vi "HandleObservationSync.vi"(8 "error in (no error)":errorcluster, 11 "S4GUI in":refnum<class "S4GUI.lvclass">) -> (0 "error out":errorcluster, 3 "S4GUI out":refnum<class "S4GUI.lvclass">)   [LabVIEW 2018, in "S4GUI.lvclass"] (continued)
          n221 = call "Read Instrument.lvclass.vi"("error in (no error)"=w570, "S4ACS_GUI in"=w571) -> ("error out"=w541:errorcluster, "Instrument.lvclass"=w542:refnum<class "Instrument.lvclass">, "S4ACS_GUI out"=w572:refnum<class "S4GUI.lvclass">)  [unwired: 7 in]
          n222 = disable-structure shown="Enabled" {
            disable-tunnel: w542 -> [w576 w589]
            disable-tunnel: w541 -> [w575 w588]
            disable-tunnel: [w574 w589] -> w540
            disable-tunnel: [w573 w588] -> w539
            frame Disabled {
              n223 = call "Read WPROT.vi"("error in (no error)"=w575, "Instrument in"=w576) -> ("error out"=w579:errorcluster, "Opt_Selector.lvclass"=w580:refnum<class "Opt_Selector.lvclass">, "Instrument out"=w586:refnum<class "Instrument.lvclass">)  [unwired: 7 in]
              n224 = call-dynamic "Read State Machine.vi"("error in (no error)"=w579, "Device in"=w580) -> ("error out"=w582:errorcluster, "State Machine.lvclass"=w584:refnum<class "State Machine.lvclass">, "Device out"=w581:refnum<class "Opt_Selector.lvclass">)  [unwired: 7 in]
              n225 = call "Next State.vi"("error in (no error)"=w582, "New_State"=30, "State Machine in"=w584) -> ("error out"=w578:errorcluster, "State Machine out"=w577:refnum<class "State Machine.lvclass">)  [unwired: 7 in]
              n226 = call-dynamic "Write State Machine.vi"("error in (no error)"=w578, "State Machine.lvclass"=w577, "Device in"=w581) -> ("error out"=w585:errorcluster, "Device out"=w587:refnum<class "Opt_Selector.lvclass">)  [unwired: 7 in]
              n227 = call "Write WPROT.vi"("error in (no error)"=w585, "Opt_Selector.lvclass"=w587, "Instrument in"=w586) -> ("error out"=w573:errorcluster, "Instrument out"=w574:refnum<class "Instrument.lvclass">)  [unwired: 7 in]
            }
            frame Enabled {
              # "depois do homing no WPSEL, o homing do WPROT é feito automaticamente pelo ICS"
            }
          }
          n228 = call "Read ASEL.vi"("error in (no error)"=w539, "Instrument in"=w540) -> ("error out"=w556:errorcluster, "Opt_Selector.lvclass"=w557:refnum<class "Opt_Selector.lvclass">, "Instrument out"=w563:refnum<class "Instrument.lvclass">)  [unwired: 7 in]
          n229 = call-dynamic "Read State Machine.vi"("error in (no error)"=w556, "Device in"=w557) -> ("error out"=w559:errorcluster, "State Machine.lvclass"=w561:refnum<class "State Machine.lvclass">, "Device out"=w558:refnum<class "Opt_Selector.lvclass">)  [unwired: 7 in]
          n230 = call "Next State.vi"("error in (no error)"=w559, "New_State"=30, "State Machine in"=w561) -> ("error out"=w555:errorcluster, "State Machine out"=w554:refnum<class "State Machine.lvclass">)  [unwired: 7 in]
          n231 = call-dynamic "Write State Machine.vi"("error in (no error)"=w555, "State Machine.lvclass"=w554, "Device in"=w558) -> ("error out"=w562:errorcluster, "Device out"=w564:refnum<class "Opt_Selector.lvclass">)  [unwired: 7 in]
          n232 = Increment(x=w565) -> (x+1=w567:u32)
          n233 = call "Write ASEL.vi"("error in (no error)"=w562, "Opt_Selector.lvclass"=w564, "Instrument in"=w563) -> ("error out"=w537:errorcluster, "Instrument out"=w538:refnum<class "Instrument.lvclass">)  [unwired: 7 in]
          n234 = call "Read GMIR.vi"("error in (no error)"=w537, "Instrument in"=w538) -> ("error out"=w545:errorcluster, "Opt_Continuous.lvclass"=w546:refnum<class "Opt_Continuous.lvclass">, "Instrument out"=w552:refnum<class "Instrument.lvclass">)  [unwired: 7 in]
          n235 = call-dynamic "Read State Machine.vi"("error in (no error)"=w545, "Device in"=w546) -> ("error out"=w548:errorcluster, "State Machine.lvclass"=w550:refnum<class "State Machine.lvclass">, "Device out"=w547:refnum<class "Opt_Continuous.lvclass">)  [unwired: 7 in]
          n236 = call "Next State.vi"("error in (no error)"=w548, "New_State"=30, "State Machine in"=w550) -> ("error out"=w544:errorcluster, "State Machine out"=w543:refnum<class "State Machine.lvclass">)  [unwired: 7 in]
          n237 = call-dynamic "Write State Machine.vi"("error in (no error)"=w544, "State Machine.lvclass"=w543, "Device in"=w547) -> ("error out"=w551:errorcluster, "Device out"=w553:refnum<class "Opt_Continuous.lvclass">)  [unwired: 7 in]
          n238 = call "Write GMIR.vi"("error in (no error)"=w551, "Opt_Continuous.lvclass"=w553, "Instrument in"=w552) -> ("error out"=w536:errorcluster, "Instrument out"=w535:refnum<class "Instrument.lvclass">)  [unwired: 7 in]
          n239 = call "Write Instrument.lvclass.vi"("error in (no error)"=w536, "Instrument.lvclass"=w535, "S4ACS_GUI in"=w572) -> ("error out"=w569:errorcluster, "S4ACS_GUI out"=w568:refnum<class "S4GUI.lvclass">)  [unwired: 7 in]
          n240 = Bundle By Name(cluster=w568, "Obs_state"=w567) -> (w566:refnum<class "S4GUI.lvclass">)
        }
        frame 223 {
          # "Espera terminar o homing de WPROT,ASEL e GFOC\nantes de seguir para o próximo estado."
          n241 = call "Read Instrument.lvclass.vi"("error in (no error)"=w614, "S4ACS_GUI in"=w615) -> ("error out"=w600:errorcluster, "Instrument.lvclass"=w601:refnum<class "Instrument.lvclass">, "S4ACS_GUI out"=w609:refnum<class "S4GUI.lvclass">)  [unwired: 7 in]
          n242 = call "Read ASEL.vi"("error in (no error)"=w600, "Instrument in"=w601) -> ("error out"=w605:errorcluster, "Opt_Selector.lvclass"=w591:refnum<class "Opt_Selector.lvclass">)  [unwired: 7 in, 1 out]
          n243 = call "Read GMIR.vi"("error in (no error)"=w600, "Instrument in"=w601) -> ("error out"=w602:errorcluster, "Opt_Continuous.lvclass"=w590:refnum<class "Opt_Continuous.lvclass">)  [unwired: 7 in, 1 out]
          n244 = disable-structure shown="Enabled" {
            disable-tunnel: [w619 w625] -> w608
            disable-tunnel: w601 -> [w618 _]
            disable-tunnel: w600 -> [w617 w625]
            disable-tunnel: [w616 0 ("State")] -> w599
            frame Disabled {
              n245 = call "Read WPROT.vi"("error in (no error)"=w617, "Instrument in"=w618) -> ("error out"=w621:errorcluster, "Opt_Selector.lvclass"=w620:refnum<class "Opt_Selector.lvclass">)  [unwired: 7 in, 1 out]
              n246 = call-dynamic "Read State Machine.vi"("error in (no error)"=w621, "Device in"=w620) -> ("error out"=w622:errorcluster, "State Machine.lvclass"=w623:refnum<class "State Machine.lvclass">)  [unwired: 7 in, 1 out]
              n247 = call-dynamic "Read State.vi"("error in (no error)"=w622, "State Machine in"=w623) -> ("error out"=w619:errorcluster, "State"=w616:i32)  [unwired: 7 in, 1 out]
            }
            frame Enabled {
            }
          }
          n248 = call-dynamic "Read State Machine.vi"("error in (no error)"=w605, "Device in"=w591) -> ("error out"=w606:errorcluster, "State Machine.lvclass"=w607:refnum<class "State Machine.lvclass">)  [unwired: 7 in, 1 out]
          n249 = call-dynamic "Read State Machine.vi"("error in (no error)"=w602, "Device in"=w590) -> ("error out"=w603:errorcluster, "State Machine.lvclass"=w604:refnum<class "State Machine.lvclass">)  [unwired: 7 in, 1 out]
          n250 = Increment(x=w611) -> (x+1=w610:u32)
          n251 = call-dynamic "Read State.vi"("error in (no error)"=w606, "State Machine in"=w607) -> ("error out"=w594:errorcluster, "State"=w598:i32)  [unwired: 7 in, 1 out]
          n252 = call-dynamic "Read State.vi"("error in (no error)"=w603, "State Machine in"=w604) -> ("error out"=w593:errorcluster, "State"=w597:i32)  [unwired: 7 in, 1 out]
          n253 = Compound Arithmetic op=ADD(w599, w598, w597) -> (w596:i32)
          n254 = Equal To 0?(x=w596) -> (x = 0?=w595:bool)
          n255 = Merge Errors(w608, w594, w593) -> (w592:errorcluster)
          n256 = Select(t=w610, s=w595, f=w611) -> (s? t:f=w612:u32)
          n257 = Bundle By Name(cluster=w609, "Obs_state"=w612) -> (w613:refnum<class "S4GUI.lvclass">)
        }
        frame 224 {
          # "40 x 0.25 = 10s"
          # "40 x 0.25 = 10s"
          # "40 x 0.25 = 10s"
          # "Manda WPSEL para OFF, CALW para OFF e ASEL para OFF"
          n258 = call "Read Instrument.lvclass.vi"("error in (no error)"=w699, "S4ACS_GUI in"=w700) -> ("error out"=w685:errorcluster, "Instrument.lvclass"=w686:refnum<class "Instrument.lvclass">, "S4ACS_GUI out"=w701:refnum<class "S4GUI.lvclass">)  [unwired: 7 in]
          n259 = call "Read WPSEL.vi"("error in (no error)"=w685, "Instrument in"=w686) -> ("error out"=w681:errorcluster, "Opt_Selector.lvclass"=w680:refnum<class "Opt_Selector.lvclass">, "Instrument out"=w693:refnum<class "Instrument.lvclass">)  [unwired: 7 in]
          n260 = call "Write target.vi"("error in (no error)"=w681, "target"=80.0, "Optics in"=w680) -> ("error out"=w684:errorcluster, "Optics out"=w679:refnum<class "Opt_Selector.lvclass">)  [unwired: 7 in]
          n261 = call "Write target name.vi"("error in (no error)"=w684, "target name"="OFF", "Optics in"=w679) -> ("error out"=w677:errorcluster, "Optics out"=w678:refnum<class "Opt_Selector.lvclass">)  [unwired: 7 in]
          n262 = call-dynamic "Read State Machine.vi"("error in (no error)"=w677, "Device in"=w678) -> ("error out"=w688:errorcluster, "State Machine.lvclass"=w690:refnum<class "State Machine.lvclass">, "Device out"=w687:refnum<class "Opt_Selector.lvclass">)  [unwired: 7 in]
          n263 = call "Next State.vi"("error in (no error)"=w688, "New_State"=1, "State Machine in"=w690) -> ("error out"=w638:errorcluster, "State Machine out"=w640:refnum<class "State Machine.lvclass">)  [unwired: 7 in]
          n264 = call-dynamic "Write Timer.vi"("error in (no error)"=w638, "Timer"=u32 40, "State Machine in"=w640) -> ("error out"=w637:errorcluster, "State Machine out"=w639:refnum<class "State Machine.lvclass">)  [unwired: 7 in]
          n265 = call-dynamic "Write State Machine.vi"("error in (no error)"=w637, "State Machine.lvclass"=w639, "Device in"=w687) -> ("error out"=w692:errorcluster, "Device out"=w694:refnum<class "Opt_Selector.lvclass">)  [unwired: 7 in]
          n266 = Increment(x=w691) -> (x+1=w696:u32)
          n267 = call "Write WPSEL.vi"("error in (no error)"=w692, "Opt_Selector.lvclass"=w694, "Instrument in"=w693) -> ("error out"=w652:errorcluster, "Instrument out"=w651:refnum<class "Instrument.lvclass">)  [unwired: 7 in]
          n268 = call "Read CALW.vi"("error in (no error)"=w652, "Instrument in"=w651) -> ("error out"=w668:errorcluster, "Opt_Selector.lvclass"=w650:refnum<class "Opt_Selector.lvclass">, "Instrument out"=w648:refnum<class "Instrument.lvclass">)  [unwired: 7 in]
          n269 = call "Write target.vi"("error in (no error)"=w668, "target"=0.0, "Optics in"=w650) -> ("error out"=w671:errorcluster, "Optics out"=w667:refnum<class "Opt_Selector.lvclass">)  [unwired: 7 in]
          n270 = call "Write target name.vi"("error in (no error)"=w671, "target name"="OFF", "Optics in"=w667) -> ("error out"=w665:errorcluster, "Optics out"=w666:refnum<class "Opt_Selector.lvclass">)  [unwired: 7 in]
          n271 = call-dynamic "Read State Machine.vi"("error in (no error)"=w665, "Device in"=w666) -> ("error out"=w673:errorcluster, "State Machine.lvclass"=w675:refnum<class "State Machine.lvclass">, "Device out"=w672:refnum<class "Opt_Selector.lvclass">)  [unwired: 7 in]
          n272 = call "Next State.vi"("error in (no error)"=w673, "New_State"=1, "State Machine in"=w675) -> ("error out"=w634:errorcluster, "State Machine out"=w635:refnum<class "State Machine.lvclass">)  [unwired: 7 in]
          n273 = call-dynamic "Write Timer.vi"("error in (no error)"=w634, "Timer"=u32 40, "State Machine in"=w635) -> ("error out"=w633:errorcluster, "State Machine out"=w632:refnum<class "State Machine.lvclass">)  [unwired: 7 in]
          n274 = call-dynamic "Write State Machine.vi"("error in (no error)"=w633, "State Machine.lvclass"=w632, "Device in"=w672) -> ("error out"=w676:errorcluster, "Device out"=w649:refnum<class "Opt_Selector.lvclass">)  [unwired: 7 in]
          n275 = call "Write CALW.vi"("error in (no error)"=w676, "Opt_Selector.lvclass"=w649, "Instrument in"=w648) -> ("error out"=w647:errorcluster, "Instrument out"=w646:refnum<class "Instrument.lvclass">)  [unwired: 7 in]
          n276 = call "Read ASEL.vi"("error in (no error)"=w647, "Instrument in"=w646) -> ("error out"=w656:errorcluster, "Opt_Selector.lvclass"=w645:refnum<class "Opt_Selector.lvclass">, "Instrument out"=w643:refnum<class "Instrument.lvclass">)  [unwired: 7 in]
          n277 = call "Write target.vi"("error in (no error)"=w656, "target"=0.0, "Optics in"=w645) -> ("error out"=w659:errorcluster, "Optics out"=w655:refnum<class "Opt_Selector.lvclass">)  [unwired: 7 in]
          n278 = call "Write target name.vi"("error in (no error)"=w659, "target name"="OFF", "Optics in"=w655) -> ("error out"=w653:errorcluster, "Optics out"=w654:refnum<class "Opt_Selector.lvclass">)  [unwired: 7 in]
          n279 = call-dynamic "Read State Machine.vi"("error in (no error)"=w653, "Device in"=w654) -> ("error out"=w661:errorcluster, "State Machine.lvclass"=w663:refnum<class "State Machine.lvclass">, "Device out"=w660:refnum<class "Opt_Selector.lvclass">)  [unwired: 7 in]
          n280 = call "Next State.vi"("error in (no error)"=w661, "New_State"=1, "State Machine in"=w663) -> ("error out"=w628:errorcluster, "State Machine out"=w629:refnum<class "State Machine.lvclass">)  [unwired: 7 in]
          n281 = call-dynamic "Write Timer.vi"("error in (no error)"=w628, "Timer"=u32 40, "State Machine in"=w629) -> ("error out"=w627:errorcluster, "State Machine out"=w626:refnum<class "State Machine.lvclass">)  [unwired: 7 in]
          n282 = call-dynamic "Write State Machine.vi"("error in (no error)"=w627, "State Machine.lvclass"=w626, "Device in"=w660) -> ("error out"=w664:errorcluster, "Device out"=w644:refnum<class "Opt_Selector.lvclass">)  [unwired: 7 in]
          n283 = call "Write ASEL.vi"("error in (no error)"=w664, "Opt_Selector.lvclass"=w644, "Instrument in"=w643) -> ("error out"=w641:errorcluster, "Instrument out"=w642:refnum<class "Instrument.lvclass">)  [unwired: 7 in]
          n284 = call "Write Instrument.lvclass.vi"("error in (no error)"=w641, "Instrument.lvclass"=w642, "S4ACS_GUI in"=w701) -> ("error out"=w698:errorcluster, "S4ACS_GUI out"=w697:refnum<class "S4GUI.lvclass">)  [unwired: 7 in]
          n285 = Bundle By Name(cluster=w697, "Obs_state"=w696) -> (w695:refnum<class "S4GUI.lvclass">)
        }
        frame 225 {
          # "Espera terminar o movimento de WPSEL, ASEL e CALW para CLEAR."
          n286 = call "Read Instrument.lvclass.vi"("error in (no error)"=w730, "S4ACS_GUI in"=w731) -> ("error out"=w713:errorcluster, "Instrument.lvclass"=w714:refnum<class "Instrument.lvclass">, "S4ACS_GUI out"=w722:refnum<class "S4GUI.lvclass">)  [unwired: 7 in]
          n287 = call "Read ASEL.vi"("error in (no error)"=w713, "Instrument in"=w714) -> ("error out"=w718:errorcluster, "Opt_Selector.lvclass"=w704:refnum<class "Opt_Selector.lvclass">)  [unwired: 7 in, 1 out]
          n288 = call "Read CALW.vi"("error in (no error)"=w713, "Instrument in"=w714) -> ("error out"=w715:errorcluster, "Opt_Selector.lvclass"=w703:refnum<class "Opt_Selector.lvclass">)  [unwired: 7 in, 1 out]
          n289 = call "Read WPSEL.vi"("error in (no error)"=w713, "Instrument in"=w714) -> ("error out"=w727:errorcluster, "Opt_Selector.lvclass"=w726:refnum<class "Opt_Selector.lvclass">)  [unwired: 7 in, 1 out]
          n290 = call-dynamic "Read State Machine.vi"("error in (no error)"=w715, "Device in"=w703) -> ("error out"=w716:errorcluster, "State Machine.lvclass"=w717:refnum<class "State Machine.lvclass">)  [unwired: 7 in, 1 out]
          n291 = call-dynamic "Read State Machine.vi"("error in (no error)"=w718, "Device in"=w704) -> ("error out"=w719:errorcluster, "State Machine.lvclass"=w720:refnum<class "State Machine.lvclass">)  [unwired: 7 in, 1 out]
          n292 = call-dynamic "Read State Machine.vi"("error in (no error)"=w727, "Device in"=w726) -> ("error out"=w728:errorcluster, "State Machine.lvclass"=w729:refnum<class "State Machine.lvclass">)  [unwired: 7 in, 1 out]
          n293 = call-dynamic "Read State.vi"("error in (no error)"=w719, "State Machine in"=w720) -> ("error out"=w707:errorcluster, "State"=w711:i32)  [unwired: 7 in, 1 out]
          n294 = call-dynamic "Read State.vi"("error in (no error)"=w716, "State Machine in"=w717) -> ("error out"=w706:errorcluster, "State"=w710:i32)  [unwired: 7 in, 1 out]
          n295 = call-dynamic "Read State.vi"("error in (no error)"=w728, "State Machine in"=w729) -> ("error out"=w721:errorcluster, "State"=w712:i32)  [unwired: 7 in, 1 out]
          n296 = Compound Arithmetic op=ADD(w712, w711, w710) -> (w709:i32)
          n297 = Equal To 0?(x=w709) -> (x = 0?=w708:bool)
          n298 = Merge Errors(w721, w707, w706) -> (w705:errorcluster)
          n299 = Select(t=u32 0, s=w708, f=w723) -> (s? t:f=w724:u32)
          n300 = Bundle By Name(cluster=w722, "Obs_state"=w724) -> (w725:refnum<class "S4GUI.lvclass">)
        }
        frame 230 {
          # "PARK:\nWPSEL = OFF\n(WPROT=NA)\nCALW=SHUTTER\nASEL=OFF"
          n301 = call "Read Instrument.lvclass.vi"("error in (no error)"=w800, "S4ACS_GUI in"=w801) -> ("error out"=w793:errorcluster, "Instrument.lvclass"=w794:refnum<class "Instrument.lvclass">, "S4ACS_GUI out"=w735:refnum<class "S4GUI.lvclass">)  [unwired: 7 in]
          n302 = call "Read WPSEL.vi"("error in (no error)"=w793, "Instrument in"=w794) -> ("error out"=w756:errorcluster, "Opt_Selector.lvclass"=w759:refnum<class "Opt_Selector.lvclass">, "Instrument out"=w789:refnum<class "Instrument.lvclass">)  [unwired: 7 in]
          n303 = call "Write target name.vi"("error in (no error)"=w756, "target name"="OFF", "Optics in"=w759) -> ("error out"=w755:errorcluster, "Optics out"=w758:refnum<class "Opt_Selector.lvclass">)  [unwired: 7 in]
          n304 = call "Write target.vi"("error in (no error)"=w755, "target"=80.0, "Optics in"=w758) -> ("error out"=w754:errorcluster, "Optics out"=w757:refnum<class "Opt_Selector.lvclass">)  [unwired: 7 in]
          n305 = call-dynamic "Read State Machine.vi"("error in (no error)"=w754, "Device in"=w757) -> ("error out"=w785:errorcluster, "State Machine.lvclass"=w787:refnum<class "State Machine.lvclass">, "Device out"=w784:refnum<class "Opt_Selector.lvclass">)  [unwired: 7 in]
          n306 = call "Next State.vi"("error in (no error)"=w785, "New_State"=1, "State Machine in"=w787) -> ("error out"=w764:errorcluster, "State Machine out"=w765:refnum<class "State Machine.lvclass">)  [unwired: 7 in]
          n307 = call-dynamic "Write State Machine.vi"("error in (no error)"=w764, "State Machine.lvclass"=w765, "Device in"=w784) -> ("error out"=w788:errorcluster, "Device out"=w790:refnum<class "Opt_Selector.lvclass">)  [unwired: 7 in]
          n308 = Increment(x=w795) -> (x+1=w797:u32)
          n309 = call "Write WPSEL.vi"("error in (no error)"=w788, "Opt_Selector.lvclass"=w790, "Instrument in"=w789) -> ("error out"=w768:errorcluster, "Instrument out"=w769:refnum<class "Instrument.lvclass">)  [unwired: 7 in]
          n310 = call "Read CALW.vi"("error in (no error)"=w768, "Instrument in"=w769) -> ("error out"=w748:errorcluster, "Opt_Selector.lvclass"=w747:refnum<class "Opt_Selector.lvclass">, "Instrument out"=w782:refnum<class "Instrument.lvclass">)  [unwired: 7 in]
          n311 = call "Write target name.vi"("error in (no error)"=w748, "target name"="SHUTTER", "Optics in"=w747) -> ("error out"=w751:errorcluster, "Optics out"=w746:refnum<class "Opt_Selector.lvclass">)  [unwired: 7 in]
          n312 = call "Write target.vi"("error in (no error)"=w751, "target"=216.0, "Optics in"=w746) -> ("error out"=w744:errorcluster, "Optics out"=w745:refnum<class "Opt_Selector.lvclass">)  [unwired: 7 in]
          n313 = call-dynamic "Read State Machine.vi"("error in (no error)"=w744, "Device in"=w745) -> ("error out"=w778:errorcluster, "State Machine.lvclass"=w780:refnum<class "State Machine.lvclass">, "Device out"=w777:refnum<class "Opt_Selector.lvclass">)  [unwired: 7 in]
          n314 = call "Next State.vi"("error in (no error)"=w778, "New_State"=1, "State Machine in"=w780) -> ("error out"=w762:errorcluster, "State Machine out"=w763:refnum<class "State Machine.lvclass">)  [unwired: 7 in]
          n315 = call-dynamic "Write State Machine.vi"("error in (no error)"=w762, "State Machine.lvclass"=w763, "Device in"=w777) -> ("error out"=w781:errorcluster, "Device out"=w783:refnum<class "Opt_Selector.lvclass">)  [unwired: 7 in]
          n316 = call "Write CALW.vi"("error in (no error)"=w781, "Opt_Selector.lvclass"=w783, "Instrument in"=w782) -> ("error out"=w766:errorcluster, "Instrument out"=w767:refnum<class "Instrument.lvclass">)  [unwired: 7 in]
          n317 = call "Read ASEL.vi"("error in (no error)"=w766, "Instrument in"=w767) -> ("error out"=w737:errorcluster, "Opt_Selector.lvclass"=w740:refnum<class "Opt_Selector.lvclass">, "Instrument out"=w775:refnum<class "Instrument.lvclass">)  [unwired: 7 in]
          n318 = call "Write target name.vi"("error in (no error)"=w737, "target name"="OFF", "Optics in"=w740) -> ("error out"=w743:errorcluster, "Optics out"=w739:refnum<class "Opt_Selector.lvclass">)  [unwired: 7 in]
          n319 = call "Write target.vi"("error in (no error)"=w743, "target"=0.0, "Optics in"=w739) -> ("error out"=w736:errorcluster, "Optics out"=w738:refnum<class "Opt_Selector.lvclass">)  [unwired: 7 in]
          n320 = call-dynamic "Read State Machine.vi"("error in (no error)"=w736, "Device in"=w738) -> ("error out"=w771:errorcluster, "State Machine.lvclass"=w773:refnum<class "State Machine.lvclass">, "Device out"=w770:refnum<class "Opt_Selector.lvclass">)  [unwired: 7 in]
          n321 = call "Next State.vi"("error in (no error)"=w771, "New_State"=1, "State Machine in"=w773) -> ("error out"=w760:errorcluster, "State Machine out"=w761:refnum<class "State Machine.lvclass">)  [unwired: 7 in]
          n322 = call-dynamic "Write State Machine.vi"("error in (no error)"=w760, "State Machine.lvclass"=w761, "Device in"=w770) -> ("error out"=w774:errorcluster, "Device out"=w776:refnum<class "Opt_Selector.lvclass">)  [unwired: 7 in]
          n323 = call "Write ASEL.vi"("error in (no error)"=w774, "Opt_Selector.lvclass"=w776, "Instrument in"=w775) -> ("error out"=w792:errorcluster, "Instrument out"=w791:refnum<class "Instrument.lvclass">)  [unwired: 7 in]
          n324 = Tick Count (ms)() -> (millisecond timer value=w732:u32)
          n325 = local write "time1"(w732) -> ()
          n326 = Bundle By Name(cluster=w735, "Error Msg"="Parking in progress. Wait....") -> (w734:refnum<class "S4GUI.lvclass">)
          n327 = call "Write Instrument.lvclass.vi"("error in (no error)"=w792, "Instrument.lvclass"=w791, "S4ACS_GUI in"=w734) -> ("error out"=w799:errorcluster, "S4ACS_GUI out"=w798:refnum<class "S4GUI.lvclass">)  [unwired: 7 in]
          n328 = Bundle By Name(cluster=w798, "Obs_state"=w797) -> (w796:refnum<class "S4GUI.lvclass">)
        }
        frame 231 {
          # "Espera terminar o parking de WPSEL,CALW e ASEL\nantes de encerrar aplicacao (exit=True)."
          n329 = call "Read Instrument.lvclass.vi"("error in (no error)"=w837, "S4ACS_GUI in"=w838) -> ("error out"=w821:errorcluster, "Instrument.lvclass"=w822:refnum<class "Instrument.lvclass">, "S4ACS_GUI out"=w830:refnum<class "S4GUI.lvclass">)  [unwired: 7 in]
          n330 = call "Read CALW.vi"("error in (no error)"=w821, "Instrument in"=w822) -> ("error out"=w826:errorcluster, "Opt_Selector.lvclass"=w812:refnum<class "Opt_Selector.lvclass">)  [unwired: 7 in, 1 out]
          n331 = call "Read ASEL.vi"("error in (no error)"=w821, "Instrument in"=w822) -> ("error out"=w823:errorcluster, "Opt_Selector.lvclass"=w811:refnum<class "Opt_Selector.lvclass">)  [unwired: 7 in, 1 out]
          n332 = call "Read WPSEL.vi"("error in (no error)"=w821, "Instrument in"=w822) -> ("error out"=w834:errorcluster, "Opt_Selector.lvclass"=w833:refnum<class "Opt_Selector.lvclass">)  [unwired: 7 in, 1 out]
          n333 = call-dynamic "Read State Machine.vi"("error in (no error)"=w826, "Device in"=w812) -> ("error out"=w827:errorcluster, "State Machine.lvclass"=w828:refnum<class "State Machine.lvclass">)  [unwired: 7 in, 1 out]
          n334 = call-dynamic "Read State Machine.vi"("error in (no error)"=w823, "Device in"=w811) -> ("error out"=w824:errorcluster, "State Machine.lvclass"=w825:refnum<class "State Machine.lvclass">)  [unwired: 7 in, 1 out]
          n335 = call-dynamic "Read State Machine.vi"("error in (no error)"=w834, "Device in"=w833) -> ("error out"=w835:errorcluster, "State Machine.lvclass"=w836:refnum<class "State Machine.lvclass">)  [unwired: 7 in, 1 out]
          n336 = Increment(x=w804) -> (x+1=w831:u32)
          n337 = call-dynamic "Read State.vi"("error in (no error)"=w827, "State Machine in"=w828) -> ("error out"=w815:errorcluster, "State"=w819:i32)  [unwired: 7 in, 1 out]
          n338 = call-dynamic "Read State.vi"("error in (no error)"=w824, "State Machine in"=w825) -> ("error out"=w814:errorcluster, "State"=w818:i32)  [unwired: 7 in, 1 out]
          n339 = call-dynamic "Read State.vi"("error in (no error)"=w835, "State Machine in"=w836) -> ("error out"=w829:errorcluster, "State"=w820:i32)  [unwired: 7 in, 1 out]
          n340 = Compound Arithmetic op=ADD(w820, w819, w818) -> (w817:i32)
          n341 = Equal To 0?(x=w817) -> (x = 0?=w816:bool)
          n342 = Merge Errors(w829, w815, w814) -> (w813:errorcluster)
          n343 = Select(t=w831, s=w816, f=w804) -> (s? t:f=w803:u32)
          n344 = Tick Count (ms)() -> (millisecond timer value=w810:u32)
          n345 = local read "time1"() -> (w808:u32)
          n346 = Subtract(x=w810, y=w808) -> (x-y=w809:u32)
          n347 = To Double Precision Float(number=w809) -> (double precision float=w807:dbl)
          n348 = Greater?(x=w807, y=30000.0) -> (0:w805:bool)
          n349 = case shown="True" w805 {
            tunnel: w804 -> [_ w841]
            tunnel: [w839 w840] -> w802
            tunnel: w803 -> [w839 _]
            frame False {
            }
            frame True {
              n350 = Increment(x=w841) -> (x+1=w840:u32)
            }
          }
          n351 = Bundle By Name(cluster=w830, "Obs_state"=w802) -> (w832:refnum<class "S4GUI.lvclass">)
        }
        frame 232 {
          n352 = Increment(x=w843) -> (x+1=w842:u32)
          n353 = Tick Count (ms)() -> (millisecond timer value=w844:u32)
          n354 = local write "time1"(w844) -> ()
          n355 = Bundle By Name(cluster=w847, "Obs_state"=w842) -> (w845:refnum<class "S4GUI.lvclass">)
        }
        frame 233 {
          # "Aguarda 1s para atualização do painel da GUI antes de encerrar..."
          n356 = local read "time1"() -> (w851:u32)
          n357 = Tick Count (ms)() -> (millisecond timer value=w852:u32)
          n358 = Subtract(x=w852, y=w851) -> (x-y=w850:u32)
          n359 = Greater?(x=w850, y=u32 1000) -> (0:w848:bool)
          n360 = case shown="True" w848 {
            tunnel: w854 -> [w858 w860]
            tunnel: [w858 w859] -> w853
            frame False {
            }
            frame True {
              n361 = Increment(x=w860) -> (x+1=w859:u32)
            }
          }
          n362 = Bundle By Name(cluster=w857, "Obs_state"=w853) -> (w855:refnum<class "S4GUI.lvclass">)
        }
        frame 234 {
          n363 = Bundle By Name(cluster=w865, "Obs_state"=u32 0, "exit"=TRUE) -> (w863:refnum<class "S4GUI.lvclass">)
        }
        frame 251 {
          # "Verifica se ha funcao valida de instrumento:"
          n364 = flat-sequence {
            tunnel: w877 -> [w1087]
            tunnel: [w1087] -> w868
            frame #0 {
              n365 = Tick Count (ms)() -> (millisecond timer value=→"time3":u32)
            }
          }
          n366 = Unbundle By Name(w874) -> ("Instrument.lvclass"=w871:refnum<class "Instrument.lvclass">)
          n367 = call-dynamic "Load Function.vi"("error in (no error)"=w868, "Instrument in"=w871) -> ("error out"=w867:errorcluster, "Instrument out"=w870:refnum<class "Instrument.lvclass">)  [unwired: 8 in]
          n368 = call-dynamic "Read Function.vi"("error in (no error)"=w867, "Instrument in"=w870) -> ("error out"=w866:errorcluster, "Function"=w872:enum16{"PHOTO", "POLAR", "NONE"}, "Instrument out"=w869:refnum<class "Instrument.lvclass">)  [unwired: 7 in]
          n369 = Bundle By Name(cluster=w874, "Instrument.lvclass"=w869) -> (w873:refnum<class "S4GUI.lvclass">)
          n370 = case shown="Default" w872 {
            tunnel: w873 -> [w886 w949]
            tunnel: w881 -> [_ w946]
            tunnel: [u32 1 ("Obs_state") w945] -> w880
            tunnel: [w885 w935] -> w879
            tunnel: [w886 w934] -> w878
            tunnel: w866 -> [w885 w933]
            tunnel: ["ERROR: No instrument function set (neither POLARIMETRICS nor PHOTOMETRICS )" ("Error Msg") w911] -> w875
            frame "NONE" {
              # "Nenhuma função valida: nem polarimetria nem fotometria..."
            }
            frame Default {
              # "POLAR ou PHOTO"
              n371 = call-dynamic "Read AcquisitionA.vi"("error in (no error)"=w933, "S4ACS_GUI in"=w949) -> ("error out"=w919:errorcluster, "Acquisition.lvclass"=w917:refnum<class "Acquisition.lvclass">, "S4ACS_GUI out"=w951:refnum<class "S4GUI.lvclass">)  [unwired: 7 in]
              n372 = call-dynamic "Read enabled.vi"("error in (no error)"=w919, "Server in"=w917) -> ("error out"=w918:errorcluster, "enabled"=w914:bool, "Server out"=w916:refnum<class "Acquisition.lvclass">)  [unwired: 7 in]
              n373 = call "Read connection.vi"("error in (no error)"=w918, "Server in"=w916) -> ("error out"=w948:errorcluster, "connection"=w920:bool, "Server out"=w947:refnum<class "Acquisition.lvclass">)  [unwired: 7 in]
              n374 = And(x=w920, y=w914) -> (x .and. y?=w915:bool)
              n375 = case shown="False" w915 {
                tunnel: [w1067 w1086] -> w952
                tunnel: [w1066 w1085] -> w950
                tunnel: w948 -> [w1066 w1084]
                tunnel: w947 -> [w1067 w1083]
                tunnel: w914 -> [w1063 _]
                tunnel: [w1062 u32 0] -> w913
                frame False {
                  n376 = Select(t=u32 1, s=w1063, f=u32 0) -> (s? t:f=w1062:u32)
                }
                frame True {
                  # "configura o canal,\nmas não dispara\na exposicao."
                  n377 = call-dynamic "Read Channel.vi"("error in (no error)"=w1084, "Acquisition in"=w1083) -> ("error out"=w1073:errorcluster, "Channel.lvclass"=w1075:refnum<class "Channel.lvclass">, "Acquisition out"=w1082:refnum<class "Acquisition.lvclass">)  [unwired: 7 in]
                  n378 = call-dynamic "Write expose.vi"("error in (no error)"=w1073, "expose"=FALSE, "Channel in"=w1075) -> ("error out"=w1072:errorcluster, "Channel out"=w1074:refnum<class "Channel.lvclass">)  [unwired: 7 in]
                  n379 = call-dynamic "Read State Machine.vi"("error in (no error)"=w1072, "Device in"=w1074) -> ("error out"=w1079:errorcluster, "State Machine.lvclass"=w1081:refnum<class "State Machine.lvclass">, "Device out"=w1077:refnum<class "Channel.lvclass">)  [unwired: 7 in]
                  n380 = call "Next State.vi"("error in (no error)"=w1079, "New_State"=1, "State Machine in"=w1081) -> ("error out"=w1069:errorcluster, "State Machine out"=w1070:refnum<class "State Machine.lvclass">)  [unwired: 7 in]
                  n381 = call-dynamic "Write State Machine.vi"("error in (no error)"=w1069, "State Machine.lvclass"=w1070, "Device in"=w1077) -> ("error out"=w1076:errorcluster, "Device out"=w1078:refnum<class "Channel.lvclass">)  [unwired: 7 in]
                  n382 = call-dynamic "Write Channel.vi"("error in (no error)"=w1076, "Channel.lvclass"=w1078, "Acquisition in"=w1082) -> ("error out"=w1085:errorcluster, "Acquisition out"=w1086:refnum<class "Acquisition.lvclass">)  [unwired: 7 in]
                }
              }
              n383 = call-dynamic "Write AcquisitionA.vi"("error in (no error)"=w950, "Acquisition.lvclass"=w952, "S4ACS_GUI in"=w951) -> ("error out"=w943:errorcluster, "S4ACS_GUI out"=w942:refnum<class "S4GUI.lvclass">)  [unwired: 7 in]
              n384 = call "Read AcquisitionB.vi"("error in (no error)"=w943, "S4ACS_GUI in"=w942) -> ("error out"=w903:errorcluster, "Acquisition.lvclass"=w905:refnum<class "Acquisition.lvclass">, "S4ACS_GUI out"=w944:refnum<class "S4GUI.lvclass">)  [unwired: 7 in]
              n385 = call-dynamic "Read enabled.vi"("error in (no error)"=w903, "Server in"=w905) -> ("error out"=w902:errorcluster, "enabled"=w887:bool, "Server out"=w904:refnum<class "Acquisition.lvclass">)  [unwired: 7 in]
              n386 = call "Read connection.vi"("error in (no error)"=w902, "Server in"=w904) -> ("error out"=w931:errorcluster, "connection"=w906:bool, "Server out"=w932:refnum<class "Acquisition.lvclass">)  [unwired: 7 in]
              n387 = And(x=w906, y=w887) -> (x .and. y?=w907:bool)
              n388 = case shown="False" w907 {
                tunnel: [w1042 w1061] -> w930
                tunnel: [w1041 w1060] -> w929
                tunnel: w931 -> [w1041 w1059]
                tunnel: w932 -> [w1042 w1058]
                tunnel: [w1038 u32 0 ("f")] -> w910
                tunnel: w887 -> [w1037 _]
                frame False {
                  n389 = Select(t=u32 2, s=w1037, f=u32 0) -> (s? t:f=w1038:u32)
                }
                frame True {
                  # "configura o canal,\nmas não dispara\na exposicao."
                  n390 = call-dynamic "Read Channel.vi"("error in (no error)"=w1059, "Acquisition in"=w1058) -> ("error out"=w1048:errorcluster, "Channel.lvclass"=w1050:refnum<class "Channel.lvclass">, "Acquisition out"=w1057:refnum<class "Acquisition.lvclass">)  [unwired: 7 in]
                  n391 = call-dynamic "Write expose.vi"("error in (no error)"=w1048, "expose"=FALSE, "Channel in"=w1050) -> ("error out"=w1047:errorcluster, "Channel out"=w1049:refnum<class "Channel.lvclass">)  [unwired: 7 in]
                  n392 = call-dynamic "Read State Machine.vi"("error in (no error)"=w1047, "Device in"=w1049) -> ("error out"=w1054:errorcluster, "State Machine.lvclass"=w1056:refnum<class "State Machine.lvclass">, "Device out"=w1052:refnum<class "Channel.lvclass">)  [unwired: 7 in]
                  n393 = call "Next State.vi"("error in (no error)"=w1054, "New_State"=1, "State Machine in"=w1056) -> ("error out"=w1044:errorcluster, "State Machine out"=w1045:refnum<class "State Machine.lvclass">)  [unwired: 7 in]
                  n394 = call-dynamic "Write State Machine.vi"("error in (no error)"=w1044, "State Machine.lvclass"=w1045, "Device in"=w1052) -> ("error out"=w1051:errorcluster, "Device out"=w1053:refnum<class "Channel.lvclass">)  [unwired: 7 in]
                  n395 = call-dynamic "Write Channel.vi"("error in (no error)"=w1051, "Channel.lvclass"=w1053, "Acquisition in"=w1057) -> ("error out"=w1060:errorcluster, "Acquisition out"=w1061:refnum<class "Acquisition.lvclass">)  [unwired: 7 in]
                }
              }
              n396 = call "Write AcquisitionB.vi"("error in (no error)"=w929, "Acquisition.lvclass"=w930, "S4ACS_GUI in"=w944) -> ("error out"=w939:errorcluster, "S4ACS_GUI out"=w938:refnum<class "S4GUI.lvclass">)  [unwired: 7 in]
              n397 = call-dynamic "Read AcquisitionC.vi"("error in (no error)"=w939, "S4ACS_GUI in"=w938) -> ("error out"=w899:errorcluster, "Acquisition.lvclass"=w901:refnum<class "Acquisition.lvclass">, "S4ACS_GUI out"=w941:refnum<class "S4GUI.lvclass">)  [unwired: 7 in]
              n398 = call-dynamic "Read enabled.vi"("error in (no error)"=w899, "Server in"=w901) -> ("error out"=w898:errorcluster, "enabled"=w888:bool, "Server out"=w900:refnum<class "Acquisition.lvclass">)  [unwired: 7 in]
              n399 = call "Read connection.vi"("error in (no error)"=w898, "Server in"=w900) -> ("error out"=w927:errorcluster, "connection"=w897:bool, "Server out"=w928:refnum<class "Acquisition.lvclass">)  [unwired: 7 in]
              n400 = And(x=w897, y=w888) -> (x .and. y?=w896:bool)
              n401 = case shown="True" w896 {
                tunnel: [w1017 w1036] -> w926
                tunnel: [w1016 w1035] -> w925
                tunnel: w927 -> [w1016 w1034]
                tunnel: w928 -> [w1017 w1033]
                tunnel: [w1013 u32 0 ("f")] -> w909
                tunnel: w888 -> [w1012 _]
                frame False {
                  n402 = Select(t=u32 4, s=w1012, f=u32 0) -> (s? t:f=w1013:u32)
                }
                frame True {
                  # "configura o canal,\nmas não dispara\na exposicao."
                  n403 = call-dynamic "Read Channel.vi"("error in (no error)"=w1034, "Acquisition in"=w1033) -> ("error out"=w1023:errorcluster, "Channel.lvclass"=w1025:refnum<class "Channel.lvclass">, "Acquisition out"=w1032:refnum<class "Acquisition.lvclass">)  [unwired: 7 in]
                  n404 = call-dynamic "Write expose.vi"("error in (no error)"=w1023, "expose"=FALSE, "Channel in"=w1025) -> ("error out"=w1022:errorcluster, "Channel out"=w1024:refnum<class "Channel.lvclass">)  [unwired: 7 in]
                  n405 = call-dynamic "Read State Machine.vi"("error in (no error)"=w1022, "Device in"=w1024) -> ("error out"=w1029:errorcluster, "State Machine.lvclass"=w1031:refnum<class "State Machine.lvclass">, "Device out"=w1027:refnum<class "Channel.lvclass">)  [unwired: 7 in]
                  n406 = call "Next State.vi"("error in (no error)"=w1029, "New_State"=1, "State Machine in"=w1031) -> ("error out"=w1019:errorcluster, "State Machine out"=w1020:refnum<class "State Machine.lvclass">)  [unwired: 7 in]
                  n407 = call-dynamic "Write State Machine.vi"("error in (no error)"=w1019, "State Machine.lvclass"=w1020, "Device in"=w1027) -> ("error out"=w1026:errorcluster, "Device out"=w1028:refnum<class "Channel.lvclass">)  [unwired: 7 in]
                  n408 = call-dynamic "Write Channel.vi"("error in (no error)"=w1026, "Channel.lvclass"=w1028, "Acquisition in"=w1032) -> ("error out"=w1035:errorcluster, "Acquisition out"=w1036:refnum<class "Acquisition.lvclass">)  [unwired: 7 in]
                }
              }
              n409 = call-dynamic "Write AcquisitionC.vi"("error in (no error)"=w925, "Acquisition.lvclass"=w926, "S4ACS_GUI in"=w941) -> ("error out"=w937:errorcluster, "S4ACS_GUI out"=w936:refnum<class "S4GUI.lvclass">)  [unwired: 7 in]
              n410 = call-dynamic "Read AcquisitionD.vi"("error in (no error)"=w937, "S4ACS_GUI in"=w936) -> ("error out"=w893:errorcluster, "Acquisition.lvclass"=w895:refnum<class "Acquisition.lvclass">, "S4ACS_GUI out"=w940:refnum<class "S4GUI.lvclass">)  [unwired: 7 in]
              n411 = call-dynamic "Read enabled.vi"("error in (no error)"=w893, "Server in"=w895) -> ("error out"=w892:errorcluster, "enabled"=w889:bool, "Server out"=w894:refnum<class "Acquisition.lvclass">)  [unwired: 7 in]
              n412 = call "Read connection.vi"("error in (no error)"=w892, "Server in"=w894) -> ("error out"=w923:errorcluster, "connection"=w891:bool, "Server out"=w924:refnum<class "Acquisition.lvclass">)  [unwired: 7 in]
              n413 = And(x=w891, y=w889) -> (x .and. y?=w890:bool)
              n414 = case shown="True" w890 {
                tunnel: [w992 w1011] -> w922
                tunnel: [w991 w1010] -> w921
                tunnel: w923 -> [w991 w1009]
                tunnel: w924 -> [w992 w1008]
                tunnel: [w988 u32 0 ("f")] -> w908
                tunnel: w889 -> [w987 _]
                frame False {
                  n415 = Select(t=u32 8, s=w987, f=u32 0) -> (s? t:f=w988:u32)
                }
                frame True {
                  # "configura o canal,\nmas não dispara\na exposicao."
                  n416 = call-dynamic "Read Channel.vi"("error in (no error)"=w1009, "Acquisition in"=w1008) -> ("error out"=w998:errorcluster, "Channel.lvclass"=w1000:refnum<class "Channel.lvclass">, "Acquisition out"=w1007:refnum<class "Acquisition.lvclass">)  [unwired: 7 in]
                  n417 = call-dynamic "Write expose.vi"("error in (no error)"=w998, "expose"=FALSE, "Channel in"=w1000) -> ("error out"=w997:errorcluster, "Channel out"=w999:refnum<class "Channel.lvclass">)  [unwired: 7 in]
                  n418 = call-dynamic "Read State Machine.vi"("error in (no error)"=w997, "Device in"=w999) -> ("error out"=w1004:errorcluster, "State Machine.lvclass"=w1006:refnum<class "State Machine.lvclass">, "Device out"=w1002:refnum<class "Channel.lvclass">)  [unwired: 7 in]
                  n419 = call "Next State.vi"("error in (no error)"=w1004, "New_State"=1, "State Machine in"=w1006) -> ("error out"=w994:errorcluster, "State Machine out"=w995:refnum<class "State Machine.lvclass">)  [unwired: 7 in]
                  n420 = call-dynamic "Write State Machine.vi"("error in (no error)"=w994, "State Machine.lvclass"=w995, "Device in"=w1002) -> ("error out"=w1001:errorcluster, "Device out"=w1003:refnum<class "Channel.lvclass">)  [unwired: 7 in]
                  n421 = call-dynamic "Write Channel.vi"("error in (no error)"=w1001, "Channel.lvclass"=w1003, "Acquisition in"=w1007) -> ("error out"=w1010:errorcluster, "Acquisition out"=w1011:refnum<class "Acquisition.lvclass">)  [unwired: 7 in]
                }
              }
              n422 = call-dynamic "Write AcquisitionD.vi"("error in (no error)"=w921, "Acquisition.lvclass"=w922, "S4ACS_GUI in"=w940) -> ("error out"=w935:errorcluster, "S4ACS_GUI out"=w934:refnum<class "S4GUI.lvclass">)  [unwired: 7 in]
              n423 = Compound Arithmetic op=ADD(w913, w910, w909, w908) -> (w912:u32)
              n424 = case shown="0, Default" w912 {
                tunnel: w946 -> [w956 _ _ _ _ _ _ _ _ _ _ _ _ _ _ _]
                tunnel: [w955 u32 1 ("Obs_state") u32 1 ("Obs_state") u32 1 ("Obs_state") u32 1 ("Obs_state") u32 1 ("Obs_state") u32 1 ("Obs_state") u32 1 ("Obs_state") u32 1 ("Obs_state") u32 1 ("Obs_state") u32 1 ("Obs_state") u32 1 ("Obs_state") u32 1 ("Obs_state") u32 1 ("Obs_state") u32 1 ("Obs_state") u32 1 ("Obs_state")] -> w945
                tunnel: ["" ("Error Msg") "ERROR: Lost channel 1 connection... - HandleObservationSync.vi state 251" ("Error Msg") "ERROR: Lost channel 2 connection...- HandleObservationSync.vi state 251" ("Error Msg") "ERROR: Lost channels 1 and 2 connection...- HandleObservationSync.vi state 251" ("Error Msg") "ERROR: Lost channel 3 connection...- HandleObservationSync.vi state 251" ("Error Msg") "ERROR: Lost channels 1 and  3 connection...- HandleObservationSync.vi state 251" ("Error Msg") "ERROR:  Lost channels 2 and  3 connection...- HandleObservationSync.vi state 251" ("Error Msg") "ERROR:  Lost channels 1, 2 and  3 connection...- HandleObservationSync.vi state 251" ("Error Msg") "ERROR: Lost channel 4 connection...- HandleObservationSync.vi state 251" ("Error Msg") "ERROR:  Lost channels 1 and 4 connection...- HandleObservationSync.vi state 251" ("Error Msg") "ERROR:  Lost channels 2 and 4 connection...- HandleObservationSync.vi state 251" ("Error Msg") "ERROR: Lost channels 1, 2 and 4 connection...- HandleObservationSync.vi state 251" ("Error Msg") "ERROR: Lost channels 3 and 4 connection...- HandleObservationSync.vi state 251" ("Error Msg") "ERROR: Lost channels 1, 3 and 4 connection...- HandleObservationSync.vi state 251" ("Error Msg") "ERROR: Lost channels 2, 3 and 4 connection...- HandleObservationSync.vi state 251" ("Error Msg") "ERROR: Lost channels 1, 2, 3 and 4 connection...- HandleObservationSync.vi state 251" ("Error Msg")] -> w911
                frame 0, Default {
                  n425 = Tick Count (ms)() -> (millisecond timer value=→"time307":u32)
                  n426 = Increment(x=w956) -> (x+1=w955:u32)
                }
                frame 1 {
                }
                frame 2 {
                }
                frame 3 {
                }
                frame 4 {
                }
                frame 5 {
                }
                frame 6 {
                }
                frame 7 {
                }
                frame 8 {
                }
                frame 9 {
                }
                frame 10 {
                }
                frame 11 {
                }
                frame 12 {
                }
                frame 13 {
                }
                frame 14 {
                }
                frame 15 {
                }
              }
            }
          }
          n427 = Bundle By Name(cluster=w878, "Obs_state"=w880, "cyclesDone"=u32 0, "Error Msg"=w875) -> (w882:refnum<class "S4GUI.lvclass">)
        }
        frame 252 {
          w1111 = 38 ("x")
          w1114 = 28 ("x")
          # "Se algum canal foi pra 38: Texp inválido \npara a configuração do CCD."
          # "Se algum canal foi pra 28: ERRO na inicialização."
          # "Espera terminar a execução da preparação\ndos 4 canais antes de ir ao proximo passo \nda Observação. E verifica se há pelo menos\n 1 canal habilitado."
          n428 = flat-sequence {
            tunnel: w1143 -> [w1288]
            tunnel: [w1288] -> w1142
            frame #0 {
              n429 = Tick Count (ms)() -> (millisecond timer value=→"time4":u32)
            }
          }
          n430 = call-dynamic "Read AcquisitionA.vi"("error in (no error)"=w1142, "S4ACS_GUI in"=w1152) -> ("error out"=w1140:errorcluster, "Acquisition.lvclass"=w1141:refnum<class "Acquisition.lvclass">, "S4ACS_GUI out"=w1154:refnum<class "S4GUI.lvclass">)  [unwired: 7 in]
          n431 = call "Read connection.vi"("error in (no error)"=w1140, "Server in"=w1141) -> ("error out"=w1138:errorcluster, "connection"=w1137:bool, "Server out"=w1139:refnum<class "Acquisition.lvclass">)  [unwired: 7 in]
          n432 = case shown="True" w1137 {
            tunnel: w1139 -> [w1271 w1287]
            tunnel: w1138 -> [w1270 w1286]
            tunnel: [w1271 w1284] -> w1155
            tunnel: [w1270 w1283] -> w1153
            tunnel: [0 ("State") w1273] -> w1110
            frame False {
            }
            frame True {
              n433 = call-dynamic "Read Channel.vi"("error in (no error)"=w1286, "Acquisition in"=w1287) -> ("error out"=w1282:errorcluster, "Channel.lvclass"=w1281:refnum<class "Channel.lvclass">, "Acquisition out"=w1285:refnum<class "Acquisition.lvclass">)  [unwired: 7 in]
              n434 = call-dynamic "Read State Machine.vi"("error in (no error)"=w1282, "Device in"=w1281) -> ("error out"=w1275:errorcluster, "State Machine.lvclass"=w1277:refnum<class "State Machine.lvclass">, "Device out"=w1279:refnum<class "Channel.lvclass">)  [unwired: 7 in]
              n435 = call-dynamic "Read State.vi"("error in (no error)"=w1275, "State Machine in"=w1277) -> ("error out"=w1274:errorcluster, "State"=w1273:i32, "State Machine out"=w1276:refnum<class "State Machine.lvclass">)  [unwired: 7 in]
              n436 = call-dynamic "Write State Machine.vi"("error in (no error)"=w1274, "State Machine.lvclass"=w1276, "Device in"=w1279) -> ("error out"=w1278:errorcluster, "Device out"=w1280:refnum<class "Channel.lvclass">)  [unwired: 7 in]
              n437 = call-dynamic "Write Channel.vi"("error in (no error)"=w1278, "Channel.lvclass"=w1280, "Acquisition in"=w1285) -> ("error out"=w1283:errorcluster, "Acquisition out"=w1284:refnum<class "Acquisition.lvclass">)  [unwired: 7 in]
            }
          }
          n438 = call-dynamic "Write AcquisitionA.vi"("error in (no error)"=w1153, "Acquisition.lvclass"=w1155, "S4ACS_GUI in"=w1154) -> ("error out"=w1149:errorcluster, "S4ACS_GUI out"=w1148:refnum<class "S4GUI.lvclass">)  [unwired: 7 in]
          n439 = call "Read AcquisitionB.vi"("error in (no error)"=w1149, "S4ACS_GUI in"=w1148) -> ("error out"=w1132:errorcluster, "Acquisition.lvclass"=w1135:refnum<class "Acquisition.lvclass">, "S4ACS_GUI out"=w1136:refnum<class "S4GUI.lvclass">)  [unwired: 7 in]
          n440 = call "Read connection.vi"("error in (no error)"=w1132, "Server in"=w1135) -> ("error out"=w1131:errorcluster, "connection"=w1133:bool, "Server out"=w1134:refnum<class "Acquisition.lvclass">)  [unwired: 7 in]
          n441 = case shown="True" w1133 {
            tunnel: w1134 -> [w1253 w1269]
            tunnel: w1131 -> [w1252 w1268]
            tunnel: [w1253 w1266] -> w1130
            tunnel: [w1252 w1265] -> w1129
            tunnel: [0 ("State") w1255] -> w1109
            frame False {
            }
            frame True {
              n442 = call-dynamic "Read Channel.vi"("error in (no error)"=w1268, "Acquisition in"=w1269) -> ("error out"=w1264:errorcluster, "Channel.lvclass"=w1263:refnum<class "Channel.lvclass">, "Acquisition out"=w1267:refnum<class "Acquisition.lvclass">)  [unwired: 7 in]
              n443 = call-dynamic "Read State Machine.vi"("error in (no error)"=w1264, "Device in"=w1263) -> ("error out"=w1257:errorcluster, "State Machine.lvclass"=w1259:refnum<class "State Machine.lvclass">, "Device out"=w1261:refnum<class "Channel.lvclass">)  [unwired: 7 in]
              n444 = call-dynamic "Read State.vi"("error in (no error)"=w1257, "State Machine in"=w1259) -> ("error out"=w1256:errorcluster, "State"=w1255:i32, "State Machine out"=w1258:refnum<class "State Machine.lvclass">)  [unwired: 7 in]
              n445 = call-dynamic "Write State Machine.vi"("error in (no error)"=w1256, "State Machine.lvclass"=w1258, "Device in"=w1261) -> ("error out"=w1260:errorcluster, "Device out"=w1262:refnum<class "Channel.lvclass">)  [unwired: 7 in]
              n446 = call-dynamic "Write Channel.vi"("error in (no error)"=w1260, "Channel.lvclass"=w1262, "Acquisition in"=w1267) -> ("error out"=w1265:errorcluster, "Acquisition out"=w1266:refnum<class "Acquisition.lvclass">)  [unwired: 7 in]
            }
          }
          n447 = call "Write AcquisitionB.vi"("error in (no error)"=w1129, "Acquisition.lvclass"=w1130, "S4ACS_GUI in"=w1136) -> ("error out"=w1147:errorcluster, "S4ACS_GUI out"=w1146:refnum<class "S4GUI.lvclass">)  [unwired: 7 in]
          n448 = call-dynamic "Read AcquisitionC.vi"("error in (no error)"=w1147, "S4ACS_GUI in"=w1146) -> ("error out"=w1127:errorcluster, "Acquisition.lvclass"=w1128:refnum<class "Acquisition.lvclass">, "S4ACS_GUI out"=w1151:refnum<class "S4GUI.lvclass">)  [unwired: 7 in]
          n449 = call "Read connection.vi"("error in (no error)"=w1127, "Server in"=w1128) -> ("error out"=w1126:errorcluster, "connection"=w1124:bool, "Server out"=w1125:refnum<class "Acquisition.lvclass">)  [unwired: 7 in]
          n450 = case shown="True" w1124 {
            tunnel: w1125 -> [w1235 w1251]
            tunnel: w1126 -> [w1234 w1250]
            tunnel: [w1235 w1248] -> w1123
            tunnel: [w1234 w1247] -> w1122
            tunnel: [0 ("State") w1237] -> w1108
            frame False {
            }
            frame True {
              n451 = call-dynamic "Read Channel.vi"("error in (no error)"=w1250, "Acquisition in"=w1251) -> ("error out"=w1246:errorcluster, "Channel.lvclass"=w1245:refnum<class "Channel.lvclass">, "Acquisition out"=w1249:refnum<class "Acquisition.lvclass">)  [unwired: 7 in]
              n452 = call-dynamic "Read State Machine.vi"("error in (no error)"=w1246, "Device in"=w1245) -> ("error out"=w1239:errorcluster, "State Machine.lvclass"=w1241:refnum<class "State Machine.lvclass">, "Device out"=w1243:refnum<class "Channel.lvclass">)  [unwired: 7 in]
              n453 = call-dynamic "Read State.vi"("error in (no error)"=w1239, "State Machine in"=w1241) -> ("error out"=w1238:errorcluster, "State"=w1237:i32, "State Machine out"=w1240:refnum<class "State Machine.lvclass">)  [unwired: 7 in]
              n454 = call-dynamic "Write State Machine.vi"("error in (no error)"=w1238, "State Machine.lvclass"=w1240, "Device in"=w1243) -> ("error out"=w1242:errorcluster, "Device out"=w1244:refnum<class "Channel.lvclass">)  [unwired: 7 in]
              n455 = call-dynamic "Write Channel.vi"("error in (no error)"=w1242, "Channel.lvclass"=w1244, "Acquisition in"=w1249) -> ("error out"=w1247:errorcluster, "Acquisition out"=w1248:refnum<class "Acquisition.lvclass">)  [unwired: 7 in]
            }
          }
          n456 = call-dynamic "Write AcquisitionC.vi"("error in (no error)"=w1122, "Acquisition.lvclass"=w1123, "S4ACS_GUI in"=w1151) -> ("error out"=w1145:errorcluster, "S4ACS_GUI out"=w1144:refnum<class "S4GUI.lvclass">)  [unwired: 7 in]
          n457 = call-dynamic "Read AcquisitionD.vi"("error in (no error)"=w1145, "S4ACS_GUI in"=w1144) -> ("error out"=w1119:errorcluster, "Acquisition.lvclass"=w1121:refnum<class "Acquisition.lvclass">, "S4ACS_GUI out"=w1150:refnum<class "S4GUI.lvclass">)  [unwired: 7 in]
          n458 = call "Read connection.vi"("error in (no error)"=w1119, "Server in"=w1121) -> ("error out"=w1118:errorcluster, "connection"=w1117:bool, "Server out"=w1120:refnum<class "Acquisition.lvclass">)  [unwired: 7 in]
          n459 = case shown="True" w1117 {
            tunnel: w1120 -> [w1217 w1233]
            tunnel: w1118 -> [w1216 w1232]
            tunnel: [w1217 w1230] -> w1116
            tunnel: [w1216 w1229] -> w1115
            tunnel: [0 ("State") w1219] -> w1107
            frame False {
            }
            frame True {
              n460 = call-dynamic "Read Channel.vi"("error in (no error)"=w1232, "Acquisition in"=w1233) -> ("error out"=w1228:errorcluster, "Channel.lvclass"=w1227:refnum<class "Channel.lvclass">, "Acquisition out"=w1231:refnum<class "Acquisition.lvclass">)  [unwired: 7 in]
              n461 = call-dynamic "Read State Machine.vi"("error in (no error)"=w1228, "Device in"=w1227) -> ("error out"=w1221:errorcluster, "State Machine.lvclass"=w1223:refnum<class "State Machine.lvclass">, "Device out"=w1225:refnum<class "Channel.lvclass">)  [unwired: 7 in]
              n462 = call-dynamic "Read State.vi"("error in (no error)"=w1221, "State Machine in"=w1223) -> ("error out"=w1220:errorcluster, "State"=w1219:i32, "State Machine out"=w1222:refnum<class "State Machine.lvclass">)  [unwired: 7 in]
              n463 = call-dynamic "Write State Machine.vi"("error in (no error)"=w1220, "State Machine.lvclass"=w1222, "Device in"=w1225) -> ("error out"=w1224:errorcluster, "Device out"=w1226:refnum<class "Channel.lvclass">)  [unwired: 7 in]
              n464 = call-dynamic "Write Channel.vi"("error in (no error)"=w1224, "Channel.lvclass"=w1226, "Acquisition in"=w1231) -> ("error out"=w1229:errorcluster, "Acquisition out"=w1230:refnum<class "Acquisition.lvclass">)  [unwired: 7 in]
            }
          }
          n465 = call-dynamic "Write AcquisitionD.vi"("error in (no error)"=w1115, "Acquisition.lvclass"=w1116, "S4ACS_GUI in"=w1150) -> ("error out"=w1101:errorcluster, "S4ACS_GUI out"=w1102:refnum<class "S4GUI.lvclass">)  [unwired: 7 in]
          n466 = Equal?(x=w1111, y=w1110) -> (x = y?=w1097:bool)
          n467 = Equal?(x=w1114, y=w1110) -> (x = y?=w1092:bool)
          n468 = Equal?(x=w1111, y=w1109) -> (x = y?=w1091:bool)
          n469 = Equal?(x=w1114, y=w1109) -> (x = y?=w1093:bool)
          n470 = Equal?(x=w1111, y=w1108) -> (x = y?=w1090:bool)
          n471 = Equal?(x=w1114, y=w1108) -> (x = y?=w1094:bool)
          n472 = Equal?(x=w1111, y=w1107) -> (x = y?=w1096:bool)
          n473 = Equal?(x=w1114, y=w1107) -> (x = y?=w1095:bool)
          n474 = call-dynamic "VerifyAcqIdle.vi"("error in (no error)"=w1101, "S4GUI in"=w1102) -> ("error out"=w1099:errorcluster, "all disabled"=w1089:bool, "idle"=w1098:bool, "S4GUI out"=w1100:refnum<class "S4GUI.lvclass">)  [unwired: 6 in]
          n475 = Compound Arithmetic op=OR(w1092, w1093, w1094, w1095) -> (w1106:bool)
          n476 = Compound Arithmetic op=OR(w1097, w1091, w1090, w1096) -> (w1105:bool)
          n477 = Build Array(w1106, w1105) -> (w1104:bool[])
          n478 = Boolean Array To Number(Boolean array=w1104) -> (number=w1103:u32)
          n479 = case shown="0, Default" w1103 {
            tunnel: w1100 -> [w1166 w1198 w1211 w1215]
            tunnel: [w1165 w1197 w1210 w1214] -> w1112
            tunnel: w1113 -> [w1167 _ _ _]
            tunnel: w1098 -> [w1163 _ _ _]
            tunnel: w1097 -> [_ _ w1208 _]
            tunnel: w1091 -> [_ _ w1207 _]
            tunnel: w1090 -> [_ _ w1206 _]
            tunnel: w1096 -> [_ _ w1205 _]
            tunnel: w1095 -> [_ w1190 _ _]
            tunnel: w1094 -> [_ w1191 _ _]
            tunnel: w1093 -> [_ w1192 _ _]
            tunnel: w1092 -> [_ w1193 _ _]
            tunnel: w1089 -> [w1156 _ _ _]
            frame 0, Default {
              n480 = local read "time307"() -> (w1161:u32)
              n481 = Tick Count (ms)() -> (millisecond timer value=w1162:u32)
              n482 = Subtract(x=w1162, y=w1161) -> (x-y=w1160:u32)
              n483 = Greater?(x=w1160, y=u32 10000) -> (0:w1158:bool)
              n484 = case shown="False" w1158 {
                tunnel: w1167 -> [w1172 _]
                tunnel: [w1171 u32 1 ("Obs_state")] -> w1164
                tunnel: w1163 -> [w1170 _]
                tunnel: [w1169 w1183] -> w1157
                tunnel: w1156 -> [w1168 _]
                frame False {
                  n485 = case shown="True" w1168 {
                    tunnel: w1172 -> [w1176 _]
                    tunnel: [w1175 u32 1 ("Obs_state")] -> w1171
                    tunnel: w1170 -> [w1174 _]
                    tunnel: ["" "ERROR: No channel enabled."] -> w1169
                    frame False {
                      # "At least 1 channel enabled."
                      n486 = disable-structure shown="Enabled" {
                        disable-tunnel: [299 ("t") 300] -> w1177
                        frame Disabled {
                        }
                        frame Enabled {
                        }
                      }
                      n487 = Select(t=w1177, s=w1174, f=w1176) -> (s? t:f=w1175:u32)
                    }
                    frame True {
                      # "No channel enabled"
                    }
                  }
                }
                frame True {
                  n488 = Concatenate Strings("CHANNEL ERROR " ("string"), ": Not idle. S4GUI:HandleObservationSync.vi state 252." ("Error Msg")) -> (w1183:string)
                }
              }
              n489 = Bundle By Name(cluster=w1166, "Obs_state"=w1164, "Error Msg"=w1157) -> (w1165:refnum<class "S4GUI.lvclass">)
            }
            frame 1 {
